vi "SpinCoaterArray2String.vi"(4 "Program Spin Coater\nSpeed (rpm)          Time (s)":dbl[][](array[numeric])) -> (1 "remote control String":string)   [LabVIEW 2020]
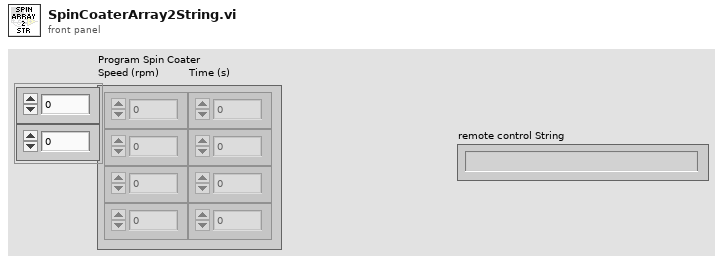
[diagram p1: front panel]
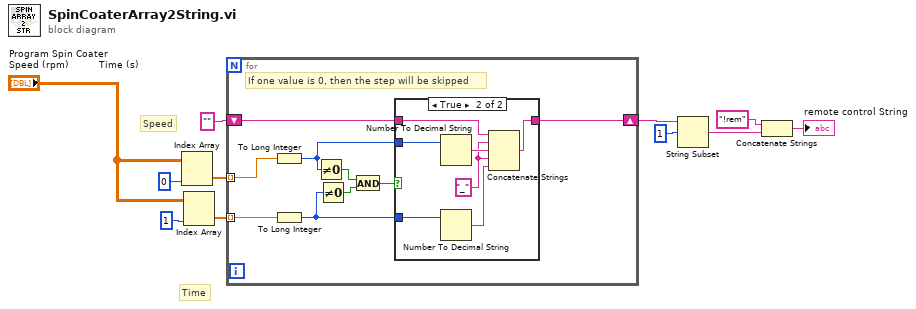
[diagram p0: block diagram]
diagram:
  # "Time"
  # "Speed"
  n1 = Index Array(array="Program Spin Coater\nSpeed (rpm)          Time (s)", index (col)=0 ("disabled index (col)")) -> (element=w8:dbl[])  [unwired: 1 in]
  n2 = Index Array(array="Program Spin Coater\nSpeed (rpm)          Time (s)", index (col)=1 ("disabled index (col)")) -> (element=w7:dbl[])  [unwired: 1 in]
  n3 = for {
    tunnel: w8 -> [w17] mode=indexing
    tunnel: w7 -> [w16] mode=indexing
    shift-right: [w12] -> w5
    shift-left: "" ("string") -> [w13]
    # "If one value is 0, then the step will be skipped"
    n4 = To Long Integer(number=w17) -> (32bit integer=w15:i32)
    n5 = To Long Integer(number=w16) -> (32bit integer=w14:i32)
    n6 = Not Equal To 0?(x=w15) -> (x != 0?=w20:bool)
    n7 = Not Equal To 0?(x=w14) -> (x != 0?=w19:bool)
    n8 = And(x=w20, y=w19) -> (x .and. y?=w18:bool)
    n9 = case shown="True" w18 {
      tunnel: w15 -> [_ w28]
      tunnel: w14 -> [_ w27]
      tunnel: w13 -> [w21 w23]
      tunnel: [w21 w22] -> w12
      frame False {
      }
      frame True {
        w24 = "_" ("string")
        n10 = Number To Decimal String(number=w28) -> (decimal integer string=w26:string)  [unwired: 1 in]
        n11 = Number To Decimal String(number=w27) -> (decimal integer string=w25:string)  [unwired: 1 in]
        n12 = Concatenate Strings(w23, w24, w26, w24, w25) -> (w22:string)
      }
    }
  }
  n13 = String Subset(string=w5, offset (0)=1) -> (substring=w2:string)  [unwired: 1 in]
  n14 = Concatenate Strings("!rem" ("string"), w2) -> (→"remote control String":string)
